vi "Test parallel sleep.vi"() -> ()   [LabVIEW 2021]
uses:
  <vilib>/Utility/RT CPU Load.ctl
  <vilib>/Platform/TimedLoop/XDataNode/timing_clust.ctl
  <vilib>/Platform/TimedLoop/XDataNode/nitl_modes.ctl
  <vilib>/Platform/TimedLoop/XDataNode/wakeup.ctl
  CIFUtilities/Time/LabVIEW Time to UTC Time.vi
  Typedef/Error Global.vi
  <vilib>/platform/TimedLoop/XDataNode/XDataNode.xnode
  CIFClocks.lvlib
  <vilib>/NI_Real-Time Target Support.lvlib
  <vilib>/Platform/TimedLoop/XDataNode/XDNodeRunTimeDep.lvlib
panel:
  out "CPU loads":T1[](array[typedef]) {"ISR (%)" format="%#.2f"; "Idle (%)" format="%#.2f"; "Background (%)" format="%#.2f"; "Normal (%)" format="%#.2f"; "Above Normal (%)" format="%#.2f"; "High (%)" format="%#.2g"; "Timed Structures (%)" format="%#.2g"; "Time Critical (%)" format="%#.2g"; "Total (%)" format="%#.2g"}
  out "appended array":T2(array[cluster])
  in  "stop":bool
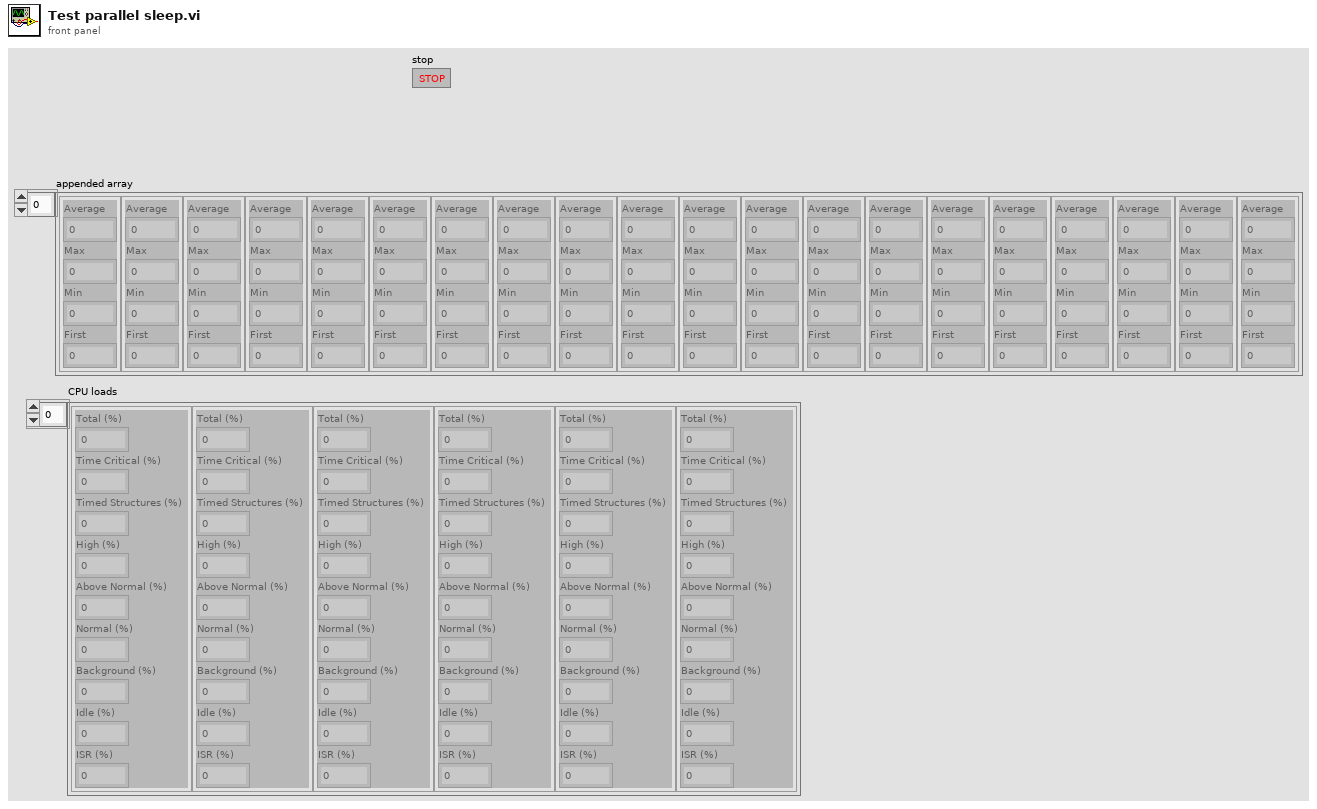
[diagram p1: front panel]
types:
  T1 = typedef "NI_Real-Time Target Support.lvlib/RT CPU Load.ctl" = cluster{"Total (%)":dbl, "Time Critical (%)":dbl, "Timed Structures (%)":dbl, "High (%)":dbl, "Above Normal (%)":dbl, "Normal (%)":dbl, "Background (%)":dbl, "Idle (%)":dbl, "ISR (%)":dbl}
  T2 = cluster{"Average":dbl, "Max":dbl, "Min":dbl, "First":dbl}[]
  T3 = typedef "XDNodeRunTimeDep.lvlib/timing_clust.ctl" = cluster{"Expected End [f-1]":u64, "Actual End [f-1]":u64, "Finished Late? [f-1]":bool, "Expected End [i-1]":u64, "Actual End [i-1]":u64, "Finished Late? [i-1]":bool, "Expected Start [i]":u64, "Actual Start [i]":u64, "Expected Start [f]":u64, "Actual Start [f]":u64, "Source Name":string, "Structure Name":string, "Period":i64, "Deadline":i64, "Offset":i64, "Start":i64, "Priority":i32, "Timeout":i32, "Mode":T4, "Wakeup Reason":T5, "Error":errorcluster, "Source Type":string, "Secondary Source Type":string, "Global End Time":u64, "Global Start Time":u64, "Frame Duration":u64, "Iteration Duration":u64, "Assigned CPU":i32, "I/O Scan Engine Mode":u32}
  T4 = typedef "XDNodeRunTimeDep.lvlib/nitl_modes.ctl" = enum32{"No Change", "Process missed periods, maintain original phase", "Discard missed periods, maintain original phase", "Process missed periods, ignore original phase", "Discard missed periods, ignore original phase"}
  T5 = typedef "XDNodeRunTimeDep.lvlib/wakeup.ctl" = enum32{"Normal", "Aborted", "Asynchronous wakeup", "Timing source error", "Timed loop error", "Timeout"}
  T6 = cluster{"Average":dbl, "Max":dbl, "Min":dbl, "First":dbl}
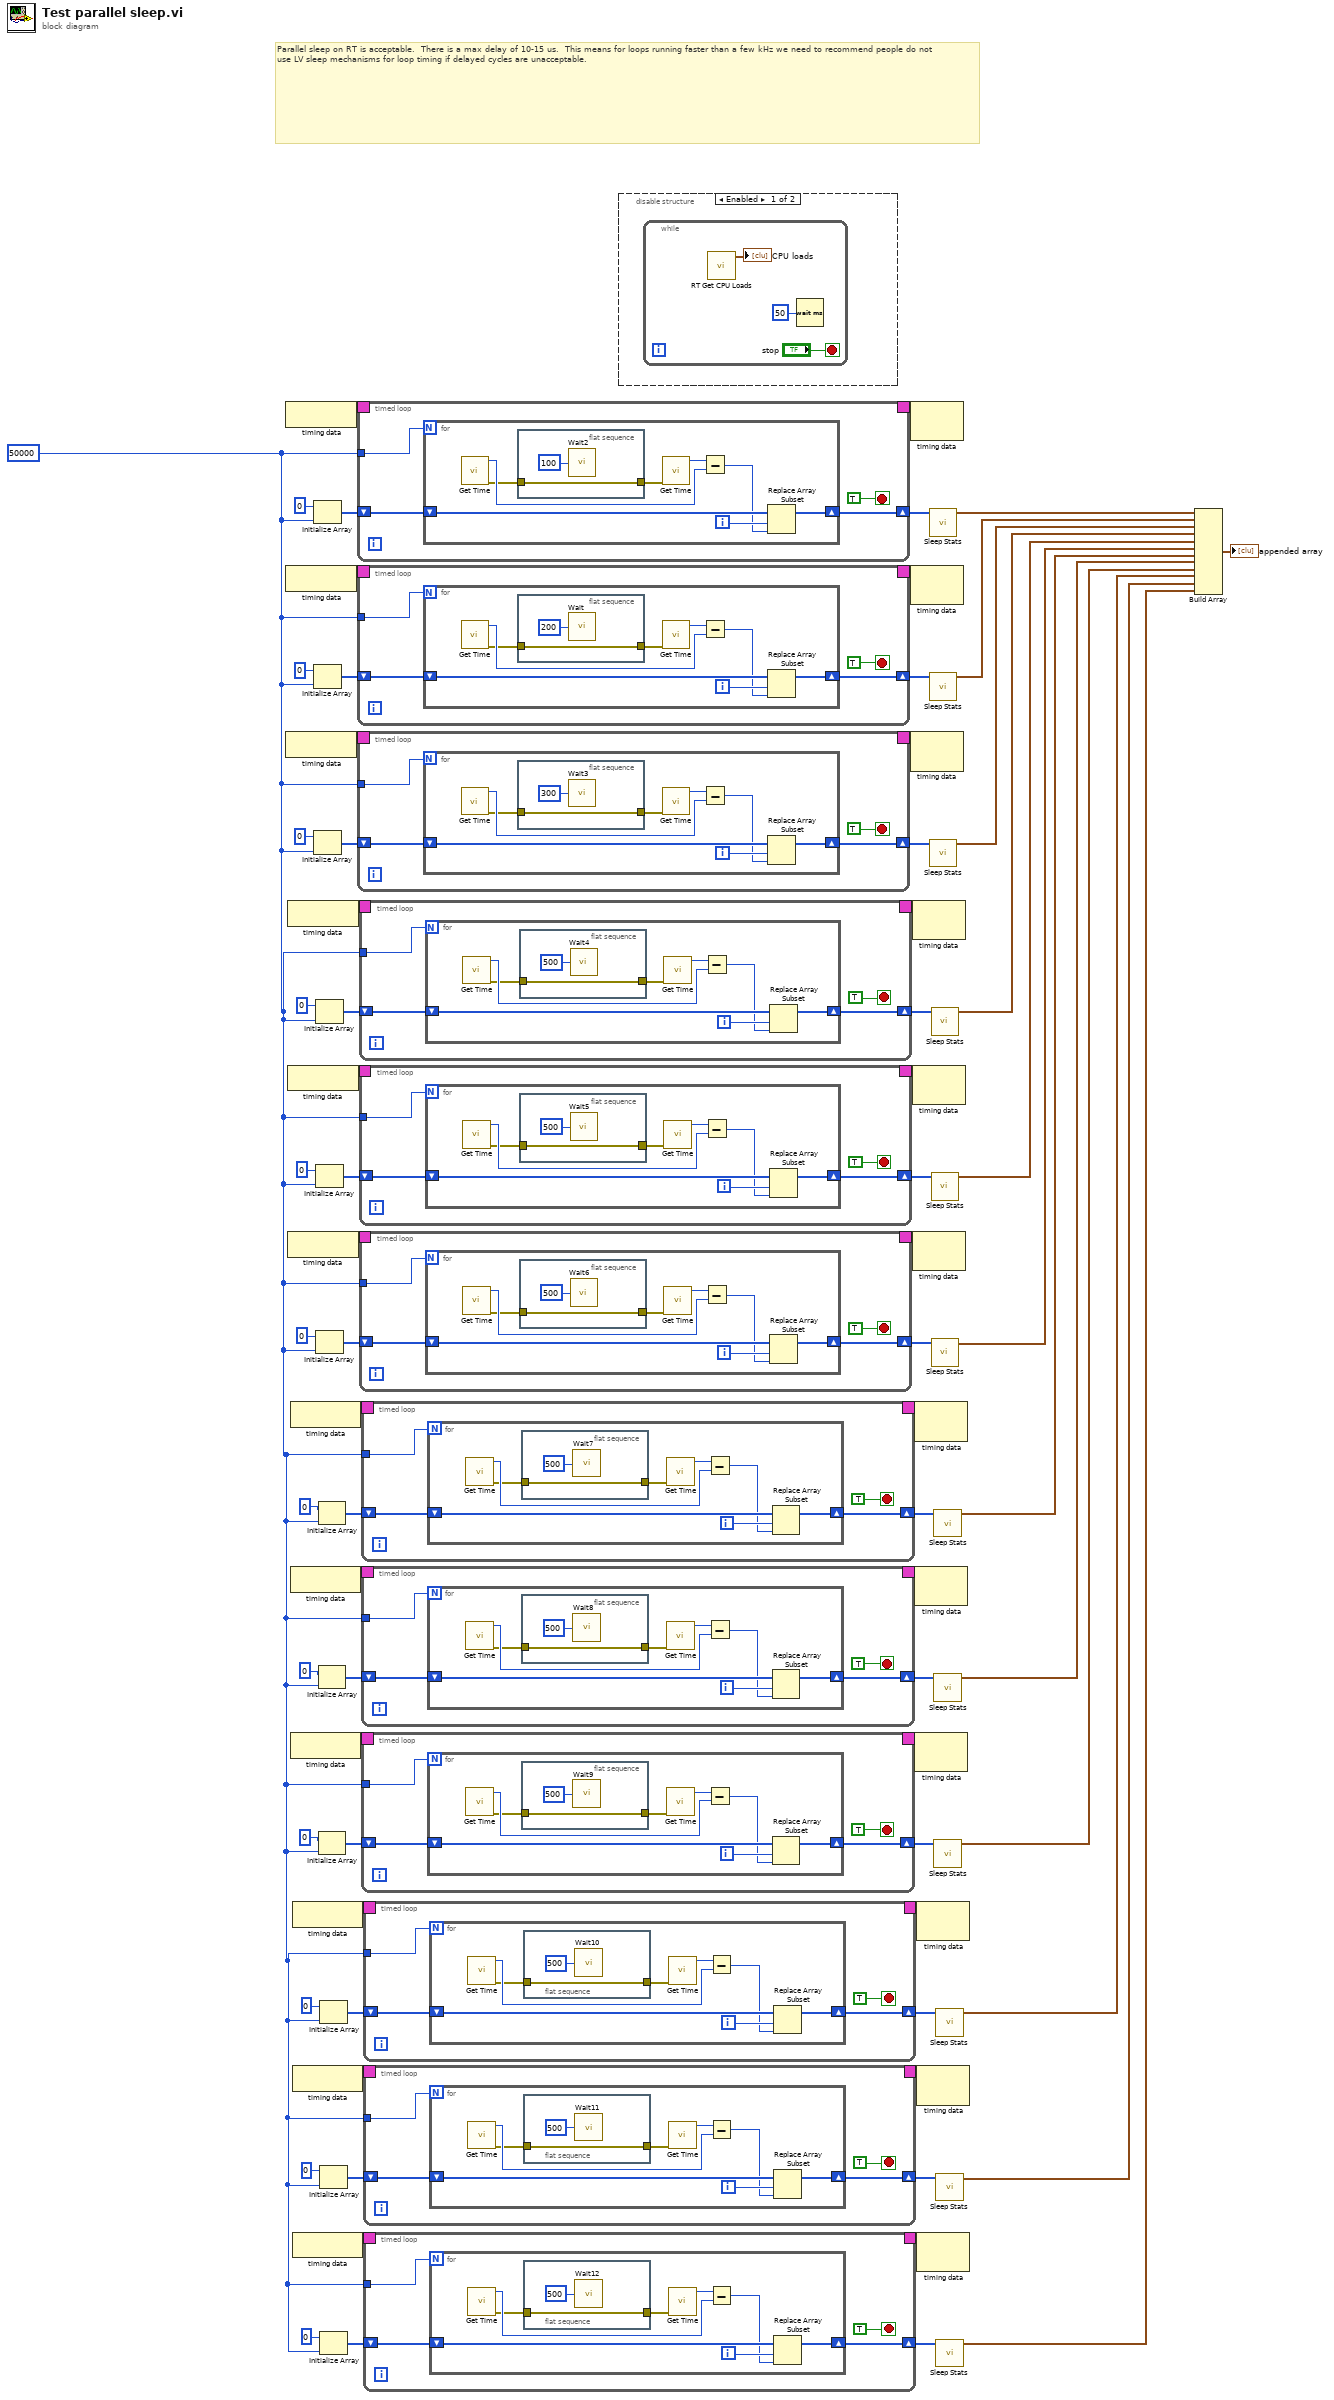
[diagram p0: block diagram]
diagram:
  w39 = 50000
  # "Parallel sleep on RT is acceptable.  There is a max delay of 10-15 us.  This means for loops running faster than a few kHz we need to recommend people do not use LV sleep mechanisms for loop timing if delayed cycles are unacceptable."
  n1 = node-c288() -> (w71:T3)
  n2 = node-c288() -> (w69:T3)
  n3 = node-c288() -> (w64:T3)
  n4 = node-c288() -> (w59:T3)
  n5 = node-c288() -> (w57:T3)
  n6 = node-c288() -> (w55:T3)
  n7 = node-c288() -> (w44:T3)
  n8 = node-c288() -> (w25:T3)
  n9 = node-c288() -> (w23:T3)
  n10 = node-c288() -> (w21:T3)
  n11 = node-c288() -> (w19:T3)
  n12 = node-c288() -> (w17:T3)
  n13 = Initialize Array(u64 0, w39) -> (w73:u64[])
  n14 = Initialize Array(u64 0, w39) -> (w66:u64[])
  n15 = Initialize Array(u64 0, w39) -> (w61:u64[])
  n16 = Initialize Array(u64 0, w39) -> (w46:u64[])
  n17 = Initialize Array(u64 0, w39) -> (w49:u64[])
  n18 = Initialize Array(u64 0, w39) -> (w52:u64[])
  n19 = Initialize Array(u64 0, w39) -> (w41:u64[])
  n20 = Initialize Array(u64 0, w39) -> (w2:u64[])
  n21 = Initialize Array(u64 0, w39) -> (w5:u64[])
  n22 = Initialize Array(u64 0, w39) -> (w14:u64[])
  n23 = Initialize Array(u64 0, w39) -> (w11:u64[])
  n24 = Initialize Array(u64 0, w39) -> (w8:u64[])
  n25 = timed-loop {
    timing: w71 -> [_]
    timing-out: [_] -> w70
    tunnel: w39 -> [w78]
    shift-right: [w76] -> w72
    shift-left: w73 -> [w77]
    stop <- TRUE stop-if-true
    n26 = for {
      N: w78 -> [_]
      shift-right: [w83] -> w76
      shift-left: w77 -> [w84]
      i -> [w82]
      n27 = call "Get Time.vi"() -> ("error out"=w80:errorcluster, "Time (ns)"=w85:u64)  [unwired: 9 in, 1 out]
      n28 = flat-sequence {
        tunnel: w80 -> [w87]
        tunnel: [w87] -> w79
        frame #0 {
          n29 = call "Wait2"("Count(uSec)"=u32 100) -> ()  [unwired: 1 out]
        }
      }
      n30 = call "Get Time.vi"("error in (no error)"=w79) -> ("Time (ns)"=w86:u64)  [unwired: 8 in, 2 out]
      n31 = Subtract(x=w86, y=w85) -> (x-y=w81:u64)
      n32 = Replace Array Subset(array=w84, new element=w81, index=w82) -> (w83:u64[])
    }
  }
  n33 = timed-loop {
    timing: w69 -> [_]
    timing-out: [_] -> w68
    tunnel: w39 -> [w94]
    shift-right: [w92] -> w67
    shift-left: w66 -> [w93]
    stop <- TRUE stop-if-true
    n34 = for {
      N: w94 -> [_]
      shift-right: [w99] -> w92
      shift-left: w93 -> [w100]
      i -> [w98]
      n35 = call "Get Time.vi"() -> ("error out"=w96:errorcluster, "Time (ns)"=w101:u64)  [unwired: 9 in, 1 out]
      n36 = flat-sequence {
        tunnel: w96 -> [w103]
        tunnel: [w103] -> w95
        frame #0 {
          n37 = call "Wait"("Count(uSec)"=u32 200) -> ()  [unwired: 1 out]
        }
      }
      n38 = call "Get Time.vi"("error in (no error)"=w95) -> ("Time (ns)"=w102:u64)  [unwired: 8 in, 2 out]
      n39 = Subtract(x=w102, y=w101) -> (x-y=w97:u64)
      n40 = Replace Array Subset(array=w100, new element=w97, index=w98) -> (w99:u64[])
    }
  }
  n41 = timed-loop {
    timing: w64 -> [_]
    timing-out: [_] -> w63
    tunnel: w39 -> [w110]
    shift-right: [w108] -> w60
    shift-left: w61 -> [w109]
    stop <- TRUE stop-if-true
    n42 = for {
      N: w110 -> [_]
      shift-right: [w115] -> w108
      shift-left: w109 -> [w116]
      i -> [w114]
      n43 = call "Get Time.vi"() -> ("error out"=w112:errorcluster, "Time (ns)"=w117:u64)  [unwired: 9 in, 1 out]
      n44 = flat-sequence {
        tunnel: w112 -> [w119]
        tunnel: [w119] -> w111
        frame #0 {
          n45 = call "Wait3"("Count(uSec)"=u32 300) -> ()  [unwired: 1 out]
        }
      }
      n46 = call "Get Time.vi"("error in (no error)"=w111) -> ("Time (ns)"=w118:u64)  [unwired: 8 in, 2 out]
      n47 = Subtract(x=w118, y=w117) -> (x-y=w113:u64)
      n48 = Replace Array Subset(array=w116, new element=w113, index=w114) -> (w115:u64[])
    }
  }
  n49 = timed-loop {
    timing: w59 -> [_]
    timing-out: [_] -> w58
    tunnel: w39 -> [w126]
    shift-right: [w124] -> w47
    shift-left: w46 -> [w125]
    stop <- TRUE stop-if-true
    n50 = for {
      N: w126 -> [_]
      shift-right: [w131] -> w124
      shift-left: w125 -> [w132]
      i -> [w130]
      n51 = call "Get Time.vi"() -> ("error out"=w128:errorcluster, "Time (ns)"=w133:u64)  [unwired: 9 in, 1 out]
      n52 = flat-sequence {
        tunnel: w128 -> [w135]
        tunnel: [w135] -> w127
        frame #0 {
          n53 = call "Wait4"("Count(uSec)"=u32 500) -> ()  [unwired: 1 out]
        }
      }
      n54 = call "Get Time.vi"("error in (no error)"=w127) -> ("Time (ns)"=w134:u64)  [unwired: 8 in, 2 out]
      n55 = Subtract(x=w134, y=w133) -> (x-y=w129:u64)
      n56 = Replace Array Subset(array=w132, new element=w129, index=w130) -> (w131:u64[])
    }
  }
  n57 = timed-loop {
    timing: w57 -> [_]
    timing-out: [_] -> w56
    tunnel: w39 -> [w142]
    shift-right: [w140] -> w48
    shift-left: w49 -> [w141]
    stop <- TRUE stop-if-true
    n58 = for {
      N: w142 -> [_]
      shift-right: [w147] -> w140
      shift-left: w141 -> [w148]
      i -> [w146]
      n59 = call "Get Time.vi"() -> ("error out"=w144:errorcluster, "Time (ns)"=w149:u64)  [unwired: 9 in, 1 out]
      n60 = flat-sequence {
        tunnel: w144 -> [w151]
        tunnel: [w151] -> w143
        frame #0 {
          n61 = call "Wait5"("Count(uSec)"=u32 500) -> ()  [unwired: 1 out]
        }
      }
      n62 = call "Get Time.vi"("error in (no error)"=w143) -> ("Time (ns)"=w150:u64)  [unwired: 8 in, 2 out]
      n63 = Subtract(x=w150, y=w149) -> (x-y=w145:u64)
      n64 = Replace Array Subset(array=w148, new element=w145, index=w146) -> (w147:u64[])
    }
  }
  n65 = timed-loop {
    timing: w55 -> [_]
    timing-out: [_] -> w54
    tunnel: w39 -> [w158]
    shift-right: [w156] -> w53
    shift-left: w52 -> [w157]
    stop <- TRUE stop-if-true
    n66 = for {
      N: w158 -> [_]
      shift-right: [w163] -> w156
      shift-left: w157 -> [w164]
      i -> [w162]
      n67 = call "Get Time.vi"() -> ("error out"=w160:errorcluster, "Time (ns)"=w165:u64)  [unwired: 9 in, 1 out]
      n68 = flat-sequence {
        tunnel: w160 -> [w167]
        tunnel: [w167] -> w159
        frame #0 {
          n69 = call "Wait6"("Count(uSec)"=u32 500) -> ()  [unwired: 1 out]
        }
      }
      n70 = call "Get Time.vi"("error in (no error)"=w159) -> ("Time (ns)"=w166:u64)  [unwired: 8 in, 2 out]
      n71 = Subtract(x=w166, y=w165) -> (x-y=w161:u64)
      n72 = Replace Array Subset(array=w164, new element=w161, index=w162) -> (w163:u64[])
    }
  }
  n73 = timed-loop {
    timing: w44 -> [_]
    timing-out: [_] -> w43
    tunnel: w39 -> [w174]
    shift-right: [w172] -> w42
    shift-left: w41 -> [w173]
    stop <- TRUE stop-if-true
    n74 = for {
      N: w174 -> [_]
      shift-right: [w179] -> w172
      shift-left: w173 -> [w180]
      i -> [w178]
      n75 = call "Get Time.vi"() -> ("error out"=w176:errorcluster, "Time (ns)"=w181:u64)  [unwired: 9 in, 1 out]
      n76 = flat-sequence {
        tunnel: w176 -> [w183]
        tunnel: [w183] -> w175
        frame #0 {
          n77 = call "Wait7"("Count(uSec)"=u32 500) -> ()  [unwired: 1 out]
        }
      }
      n78 = call "Get Time.vi"("error in (no error)"=w175) -> ("Time (ns)"=w182:u64)  [unwired: 8 in, 2 out]
      n79 = Subtract(x=w182, y=w181) -> (x-y=w177:u64)
      n80 = Replace Array Subset(array=w180, new element=w177, index=w178) -> (w179:u64[])
    }
  }
  n81 = timed-loop {
    timing: w25 -> [_]
    timing-out: [_] -> w24
    tunnel: w39 -> [w190]
    shift-right: [w188] -> w1
    shift-left: w2 -> [w189]
    stop <- TRUE stop-if-true
    n82 = for {
      N: w190 -> [_]
      shift-right: [w195] -> w188
      shift-left: w189 -> [w196]
      i -> [w194]
      n83 = call "Get Time.vi"() -> ("error out"=w192:errorcluster, "Time (ns)"=w197:u64)  [unwired: 9 in, 1 out]
      n84 = flat-sequence {
        tunnel: w192 -> [w199]
        tunnel: [w199] -> w191
        frame #0 {
          n85 = call "Wait8"("Count(uSec)"=u32 500) -> ()  [unwired: 1 out]
        }
      }
      n86 = call "Get Time.vi"("error in (no error)"=w191) -> ("Time (ns)"=w198:u64)  [unwired: 8 in, 2 out]
      n87 = Subtract(x=w198, y=w197) -> (x-y=w193:u64)
      n88 = Replace Array Subset(array=w196, new element=w193, index=w194) -> (w195:u64[])
    }
  }
  n89 = timed-loop {
    timing: w23 -> [_]
    timing-out: [_] -> w22
    tunnel: w39 -> [w206]
    shift-right: [w204] -> w6
    shift-left: w5 -> [w205]
    stop <- TRUE stop-if-true
    n90 = for {
      N: w206 -> [_]
      shift-right: [w211] -> w204
      shift-left: w205 -> [w212]
      i -> [w210]
      n91 = call "Get Time.vi"() -> ("error out"=w208:errorcluster, "Time (ns)"=w213:u64)  [unwired: 9 in, 1 out]
      n92 = flat-sequence {
        tunnel: w208 -> [w215]
        tunnel: [w215] -> w207
        frame #0 {
          n93 = call "Wait9"("Count(uSec)"=u32 500) -> ()  [unwired: 1 out]
        }
      }
      n94 = call "Get Time.vi"("error in (no error)"=w207) -> ("Time (ns)"=w214:u64)  [unwired: 8 in, 2 out]
      n95 = Subtract(x=w214, y=w213) -> (x-y=w209:u64)
      n96 = Replace Array Subset(array=w212, new element=w209, index=w210) -> (w211:u64[])
    }
  }
  n97 = timed-loop {
    timing: w21 -> [_]
    timing-out: [_] -> w20
    tunnel: w39 -> [w222]
    shift-right: [w220] -> w13
    shift-left: w14 -> [w221]
    stop <- TRUE stop-if-true
    n98 = for {
      N: w222 -> [_]
      shift-right: [w227] -> w220
      shift-left: w221 -> [w228]
      i -> [w226]
      n99 = call "Get Time.vi"() -> ("error out"=w224:errorcluster, "Time (ns)"=w229:u64)  [unwired: 9 in, 1 out]
      n100 = flat-sequence {
        tunnel: w224 -> [w231]
        tunnel: [w231] -> w223
        frame #0 {
          n101 = call "Wait10"("Count(uSec)"=u32 500) -> ()  [unwired: 1 out]
        }
      }
      n102 = call "Get Time.vi"("error in (no error)"=w223) -> ("Time (ns)"=w230:u64)  [unwired: 8 in, 2 out]
      n103 = Subtract(x=w230, y=w229) -> (x-y=w225:u64)
      n104 = Replace Array Subset(array=w228, new element=w225, index=w226) -> (w227:u64[])
    }
  }
  n105 = timed-loop {
    timing: w19 -> [_]
    timing-out: [_] -> w18
    tunnel: w39 -> [w238]
    shift-right: [w236] -> w12
    shift-left: w11 -> [w237]
    stop <- TRUE stop-if-true
    n106 = for {
      N: w238 -> [_]
      shift-right: [w243] -> w236
      shift-left: w237 -> [w244]
      i -> [w242]
      n107 = call "Get Time.vi"() -> ("error out"=w240:errorcluster, "Time (ns)"=w245:u64)  [unwired: 9 in, 1 out]
      n108 = flat-sequence {
        tunnel: w240 -> [w247]
        tunnel: [w247] -> w239
        frame #0 {
          n109 = call "Wait11"("Count(uSec)"=u32 500) -> ()  [unwired: 1 out]
        }
      }
      n110 = call "Get Time.vi"("error in (no error)"=w239) -> ("Time (ns)"=w246:u64)  [unwired: 8 in, 2 out]
      n111 = Subtract(x=w246, y=w245) -> (x-y=w241:u64)
      n112 = Replace Array Subset(array=w244, new element=w241, index=w242) -> (w243:u64[])
    }
  }
  n113 = timed-loop {
    timing: w17 -> [_]
    timing-out: [_] -> w16
    tunnel: w39 -> [w254]
    shift-right: [w252] -> w7
    shift-left: w8 -> [w253]
    stop <- TRUE stop-if-true
    n114 = for {
      N: w254 -> [_]
      shift-right: [w259] -> w252
      shift-left: w253 -> [w260]
      i -> [w258]
      n115 = call "Get Time.vi"() -> ("error out"=w256:errorcluster, "Time (ns)"=w261:u64)  [unwired: 9 in, 1 out]
      n116 = flat-sequence {
        tunnel: w256 -> [w263]
        tunnel: [w263] -> w255
        frame #0 {
          n117 = call "Wait12"("Count(uSec)"=u32 500) -> ()  [unwired: 1 out]
        }
      }
      n118 = call "Get Time.vi"("error in (no error)"=w255) -> ("Time (ns)"=w262:u64)  [unwired: 8 in, 2 out]
      n119 = Subtract(x=w262, y=w261) -> (x-y=w257:u64)
      n120 = Replace Array Subset(array=w260, new element=w257, index=w258) -> (w259:u64[])
    }
  }
  n121 = disable-structure shown="Enabled" {
    frame Enabled {
      n122 = while {
        stop <- "stop" stop-if-true
        n123 = call <vilib>:"RT Get CPU Loads.vi"() -> ("CPU loads"=→"CPU loads":T1[])  [unwired: 10 in, 1 out]
        n124 = Wait (ms)(milliseconds to wait=u32 50) -> ()  [unwired: 1 out]
      }
    }
    frame Disabled {
    }
  }
  n125 = node-c288(w70) -> ()  [unwired: 1 out]
  n126 = node-c288(w68) -> ()  [unwired: 1 out]
  n127 = node-c288(w63) -> ()  [unwired: 1 out]
  n128 = node-c288(w58) -> ()  [unwired: 1 out]
  n129 = node-c288(w56) -> ()  [unwired: 1 out]
  n130 = node-c288(w54) -> ()  [unwired: 1 out]
  n131 = node-c288(w43) -> ()  [unwired: 1 out]
  n132 = node-c288(w24) -> ()  [unwired: 1 out]
  n133 = node-c288(w22) -> ()  [unwired: 1 out]
  n134 = node-c288(w20) -> ()  [unwired: 1 out]
  n135 = node-c288(w18) -> ()  [unwired: 1 out]
  n136 = node-c288(w16) -> ()  [unwired: 1 out]
  n137 = call "Sleep Stats.vi"("Sleep Timers"=w72) -> ("Stats"=w38:T6)  [unwired: 10 in]
  n138 = call "Sleep Stats.vi"("Sleep Timers"=w67) -> ("Stats"=w37:T6)  [unwired: 10 in]
  n139 = call "Sleep Stats.vi"("Sleep Timers"=w60) -> ("Stats"=w36:T6)  [unwired: 10 in]
  n140 = call "Sleep Stats.vi"("Sleep Timers"=w47) -> ("Stats"=w35:T6)  [unwired: 10 in]
  n141 = call "Sleep Stats.vi"("Sleep Timers"=w48) -> ("Stats"=w34:T6)  [unwired: 10 in]
  n142 = call "Sleep Stats.vi"("Sleep Timers"=w53) -> ("Stats"=w33:T6)  [unwired: 10 in]
  n143 = call "Sleep Stats.vi"("Sleep Timers"=w42) -> ("Stats"=w32:T6)  [unwired: 10 in]
  n144 = call "Sleep Stats.vi"("Sleep Timers"=w1) -> ("Stats"=w31:T6)  [unwired: 10 in]
  n145 = call "Sleep Stats.vi"("Sleep Timers"=w6) -> ("Stats"=w30:T6)  [unwired: 10 in]
  n146 = call "Sleep Stats.vi"("Sleep Timers"=w13) -> ("Stats"=w29:T6)  [unwired: 10 in]
  n147 = call "Sleep Stats.vi"("Sleep Timers"=w12) -> ("Stats"=w28:T6)  [unwired: 10 in]
  n148 = call "Sleep Stats.vi"("Sleep Timers"=w7) -> ("Stats"=w27:T6)  [unwired: 10 in]
  n149 = Build Array(w38, w37, w36, w35, w34, w33, w32, w31, w30, w29, w28, w27) -> (→"appended array":T2)
